vi "_YKWT500 SET AND Query.vi"(8 "error in (no error)":errorcluster, 10 "Write Data":string, 11 "VISA resource name":refnum<visa-resource-name>) -> (0 "error out":errorcluster, 1 "Data Length":i32, 2 "Read Data":string, 3 "VISA resource name out":refnum<visa-resource-name>)   [LabVIEW 2009]
doc: "Writes the string data and receives a maximum of bytes to read bytes from the specified interface connection, returning the results in Read Data."
panel:
  # "WILL READ ONLY WHEN WRITE ENDS WITH ?"
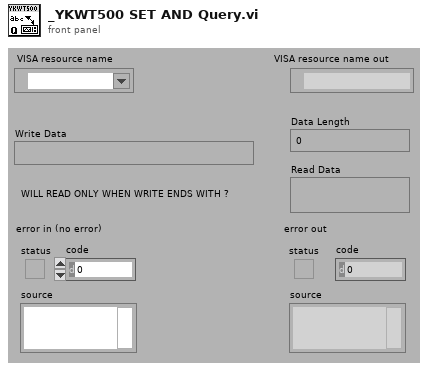
[diagram p1: front panel]
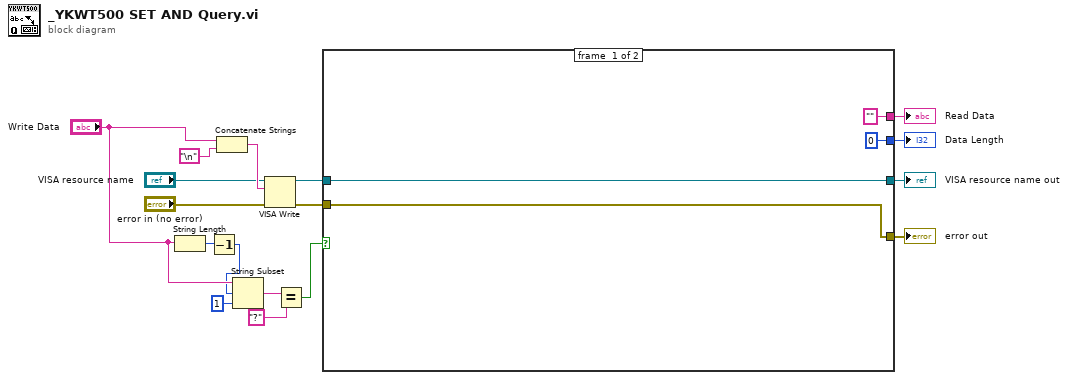
[diagram p0: block diagram]
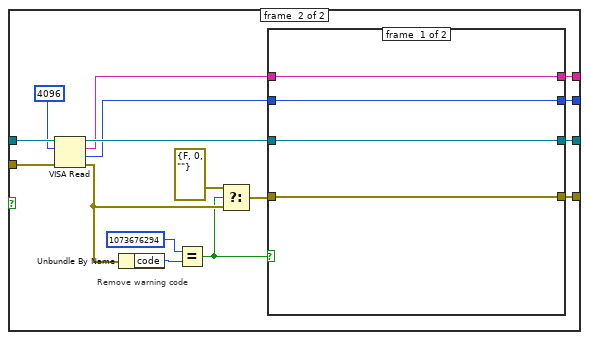
[diagram p2: hidden frame]
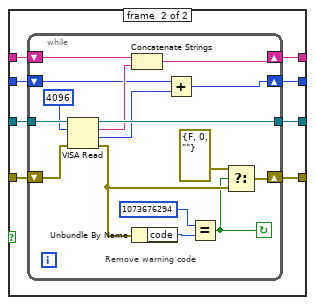
[diagram p3: hidden frame]
diagram:
  n1 = String Length(string="Write Data") -> (length=w5:i32)
  n2 = Decrement(x=w5) -> (x-1=w4:i32)
  n3 = Concatenate Strings("Write Data", "\n") -> (w12:string)
  n4 = String Subset(string="Write Data", offset (0)=w4, length (rest)=1 ("length (rest)")) -> (substring=w3:string)
  n5 = VISA Write(VISA resource name="VISA resource name", write buffer=w12, error in (no error)="error in (no error)") -> (VISA resource name out=w14:refnum<visa-resource-name>, error out=w13:errorcluster)  [unwired: 1 out]
  n6 = Equal?(x=w3, y="?") -> (x = y?=w1:bool)
  n7 = case shown="True" w1 {
    tunnel: [w20 w37] -> w17
    tunnel: [u32 0 ("return count") w36] -> w16
    tunnel: ["" ("read buffer") w35] -> w15
    tunnel: w14 -> [w20 w34]
    tunnel: w13 -> [w21 w33]
    tunnel: [w21 w22] -> w8
    frame #0 {
    }
    frame #1 {
      # "Remove warning code"
      n8 = VISA Read(VISA resource name=w34, byte count=u32 4096, error in (no error)=w33) -> (VISA resource name out=w32:refnum<visa-resource-name>, read buffer=w31:string, return count=w23:u32, error out=w26:errorcluster)
      n9 = Unbundle By Name(w26) -> ("code"=w30:i32)
      n10 = Equal?(x=1073676294, y=w30) -> (x = y?=w25:bool)
      n11 = Select(t=errorcluster {"status"=FALSE, "code"=0, "source"=""}, s=w25, f=w26) -> (s? t:f=w27:errorcluster)
      n12 = case shown="True" w25 {
        tunnel: w32 -> [w41 w49]
        tunnel: w27 -> [w40 w46]
        tunnel: [w41 w48] -> w37
        tunnel: [w40 w47] -> w22
        tunnel: w23 -> [w38 w45]
        tunnel: [w39 w44] -> w35
        tunnel: w31 -> [w39 w43]
        tunnel: [w38 w42] -> w36
        frame #0 {
        }
        frame #1 {
          n13 = while {
            shift-left: w46 -> [w60]
            shift-right: [w51] -> w47
            shift-left: w43 -> [w62]
            shift-right: [w63] -> w44
            shift-left: w45 -> [w59]
            shift-right: [w57] -> w42
            tunnel: [w64] -> w48
            tunnel: w49 -> [w65]
            stop <- w50 continue-if-true
            # "Remove warning code"
            n14 = VISA Read(VISA resource name=w65, byte count=u32 4096, error in (no error)=w60) -> (VISA resource name out=w64:refnum<visa-resource-name>, read buffer=w61:string, return count=w58:u32, error out=w52:errorcluster)
            n15 = Concatenate Strings(w62, w61) -> (w63:string)
            n16 = Unbundle By Name(w52) -> ("code"=w55:i32)
            n17 = Add(x=w59, y=w58) -> (x+y=w57:u32)
            n18 = Equal?(x=1073676294, y=w55) -> (x = y?=w50:bool)
            n19 = Select(t=errorcluster {"status"=FALSE, "code"=0, "source"=""}, s=w50, f=w52) -> (s? t:f=w51:errorcluster)
          }
        }
      }
    }
  }
  "VISA resource name out" <- w17
  "error out" <- w8
  "Data Length" <- w16
  "Read Data" <- w15
